vi "Initialization VI.vi"(8 "error in (no error)":errorcluster, 10 "Custom XML":string, 11 "Device Item Ref in":T1 format="%.0x") -> (0 "error out":errorcluster, 3 "Device Item Ref out":T1 format="%.0x")   [LabVIEW 2019, in "Instrument Addon System Explorer.lvlib"]
uses:
  Instrument Addon System Explorer.lvlib
  <vilib>/NI VeriStand/Custom Device API/Custom Device Item Ref.ctl
  Shared/Types/FG Control.ctl
  Shared/Constants.vi
  <vilib>/NI VeriStand/Custom Device API/NI VeriStand - Get Item Property.vi
  <vilib>/NI VeriStand/Custom Device API/Get Item Property (String).vi
  <vilib>/NI VeriStand/Custom Device API/NI VeriStand - Set Item Property.vi
  <vilib>/NI VeriStand/Custom Device API/Set Item Property (String).vi
  Shared/Instrument Addon Shared.lvlib
  <vilib>/NI VeriStand/Custom Device API/Custom Device API.lvlib
  <vilib>/NI/NI VeriStand Custom Device Import and Export Tool/ImportExport.lvlib
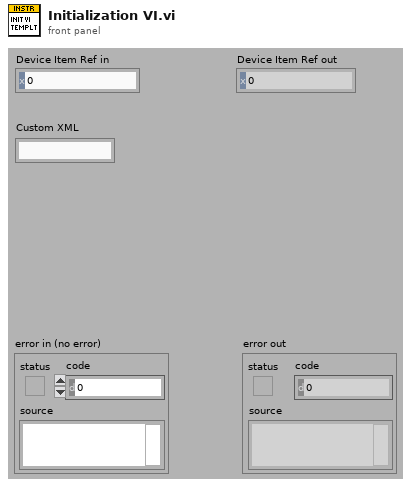
[diagram p1: front panel]
types:
  T1 = typedef "Custom Device API.lvlib/Custom Device Item Ref.ctl" = u64
  T2 = typedef "Instrument Addon Shared.lvlib/FG Control.ctl" = enum16{"Get", "Set"}
  T3 = typedef "Instrument Addon System Explorer.lvlib/Initial User Selection.ctl" = cluster{"Protocol":string}
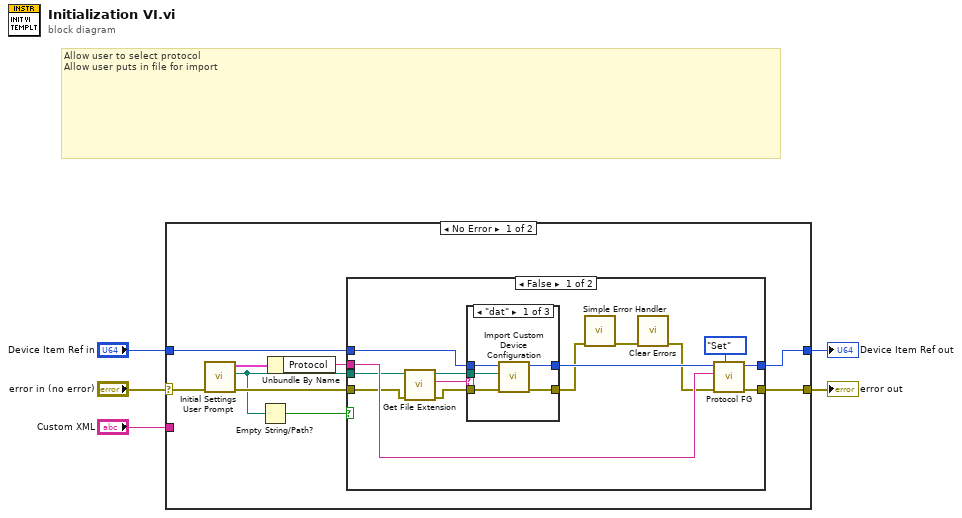
[diagram p0: block diagram]
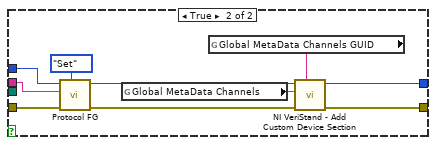
[diagram p4: hidden frame]
diagram:
  # "Allow user to select protocol\nAllow user puts in file for import"
  n1 = case shown="No Error" "error in (no error)" {
    selector: "error in (no error)" -> [w14 w48]
    tunnel: [w12 w48] -> w5
    tunnel: [w8 w47] -> w3
    tunnel: "Device Item Ref in" -> [w9 w47]
    tunnel: "Custom XML" -> [_ _]
    frame No Error {
      n2 = call "Initial Settings User Prompt.vi"("error in (no error)"=w14) -> ("error out"=w13:errorcluster, "Path out"=w6:path, "Initial Settings"=w11:T3)  [unwired: 8 in]
      n3 = Empty String/Path?(string/path=w6) -> (empty?=w7:bool)
      n4 = Unbundle By Name(w11) -> ("Protocol"=w10:string)
      n5 = case shown="False" w7 {
        tunnel: w13 -> [w17 w46]
        tunnel: [w26 w39] -> w12
        tunnel: w10 -> [w23 w40]
        tunnel: w9 -> [w28 w45]
        tunnel: [w24 w38] -> w8
        tunnel: w6 -> [w19 _]
        frame False {
          n6 = call <vilib>:"Get File Extension.vi"("error in (no error)"=w17, "file"=w19) -> ("error out"=w16:errorcluster, "lowercase file extension"=w15:string, "dup file"=w18:path)  [unwired: 5 in, 2 out]
          n7 = case shown="\"dat\"" w15 {
            tunnel: w16 -> [w32 w35 w36]
            tunnel: w28 -> [w31 w34 w37]
            tunnel: w18 -> [w29 _ _]
            tunnel: [w30 w34 w37] -> w25
            tunnel: [w33 w35 w36] -> w21
            frame "dat" {
              n8 = call <vilib>:"Import Custom Device Configuration.vi"("error in (no error)"=w32, "Path"=w29, "NodeID"=w31) -> ("error out"=w33:errorcluster, "NodeID out"=w30:u64)  [unwired: 6 in, 1 out]
            }
            frame "xml" {
            }
            frame Default {
            }
          }
          n9 = call <vilib>:"Simple Error Handler.vi"("error in (no error)"=w21) -> ("error out"=w22:errorcluster)  [unwired: 4 in, 4 out]
          n10 = call <vilib>:"Clear Errors.vi"("error in (no error)"=w22) -> ("error out"=w20:errorcluster)  [unwired: 5 in, 1 out]
          n11 = call "Protocol FG.vi"("Action"=FG_Control."Set", "error in (no error)"=w20, "Protocol"=w23, "Device Item Ref in"=w25) -> ("error out"=w26:errorcluster, "Item Ref out"=w24:T1)  [unwired: 5 in, 1 out]
        }
        frame True {
          n12 = call "Protocol FG.vi"("Action"=FG_Control."Set", "error in (no error)"=w46, "Protocol"=w40, "Device Item Ref in"=w45) -> ("error out"=w39:errorcluster, "Item Ref out"=w44:T1)  [unwired: 5 in, 1 out]
          n13 = global read "Constants.vi" "Global MetaData Channels"() -> (w41:string)
          n14 = global read "Constants.vi" "Global MetaData Channels GUID"() -> (w42:string)
          n15 = call <vilib>:"NI VeriStand - Add Custom Device Section.vi"("GUID (Default Section)"=w42, "Section Name"=w41, "Parent Ref in"=w44) -> ("Parent Ref out"=w38:T1)  [unwired: 5 in, 3 out]
        }
      }
    }
    frame Error {
    }
  }
  "error out" <- w5
  "Device Item Ref out" <- w3
